vi "SDSU_REgister2Str.vi"(9 "send comment":bool, 10 "Register":T1) -> (1 "fields info":string, 2 "full info":string)   [LabVIEW 2016]
uses:
  SDSU_Register.ctl
  SDSU_RegField.ctl
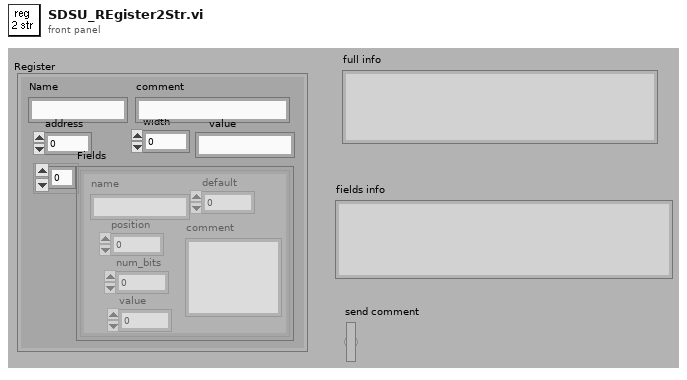
[diagram p1: front panel]
types:
  T1 = typedef "SDSU_Register.ctl" = cluster{"Name":string, "address":i16, "width":i16, "comment":string, "Fields":T2[], "value":string}
  T2 = typedef "SDSU_RegField.ctl" = cluster{"name":string, "position":u16, "num_bits":u16, "default":i16, "comment":string, "value":i32}
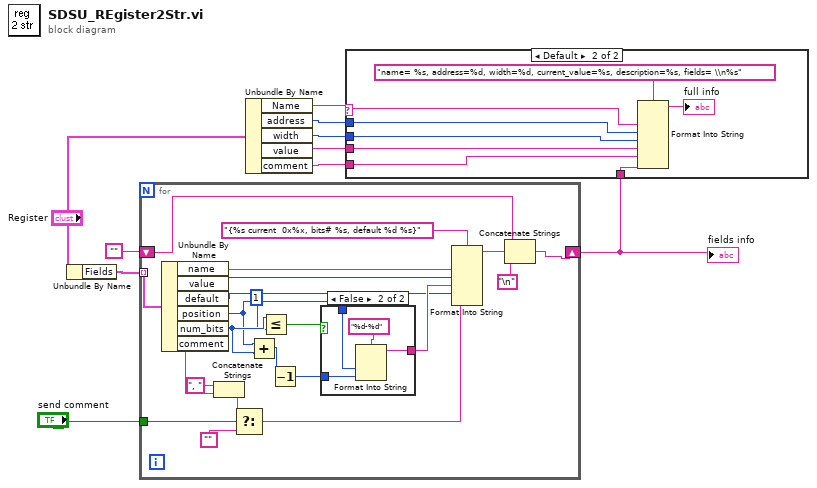
[diagram p0: block diagram]
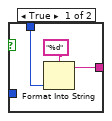
[diagram p3: hidden frame]
diagram:
  n1 = Unbundle By Name("Register") -> ("Fields"=w10:T2[])
  n2 = for {
    tunnel: w10 -> [w32] mode=indexing
    shift-right: [w27] -> w3
    shift-left: "" -> [w26]
    tunnel: "send comment" -> [w17]
    n3 = Unbundle By Name(w32) -> ("name"=w30:string, "value"=w29:i32, "default"=w20:i16, "position"=w23:u16, "num_bits"=w25:u16, "comment"=w14:string)
    n4 = Concatenate Strings(", " ("string"), w14) -> (w12:string)
    n5 = Select(t=w12, s=w17, f="") -> (s? t:f=w15:string)
    n6 = Add(x=w23, y=w25) -> (x+y=w22:u16)
    n7 = Less Or Equal?(x=w25, y=u16 1) -> (x <= y?=w19:bool)
    n8 = Decrement(x=w22) -> (x-1=w11:u16)
    n9 = case shown="False" w19 {
      tunnel: w23 -> [w35 w39]
      tunnel: w11 -> [_ w38]
      tunnel: [w34 w37] -> w21
      frame True {
        n10 = Format Into String(format string="%d", w35) -> (resulting string=w34:string)  [unwired: 2 in, 1 out]
      }
      frame False {
        n11 = Format Into String(format string="%d-%d", w39, w38) -> (resulting string=w37:string)  [unwired: 2 in, 1 out]
      }
    }
    n12 = Format Into String(format string="{%s current  0x%x, bits# %s, default %d %s}", w30, w29, w21, w20, w15) -> (resulting string=w28:string)  [unwired: 2 in, 1 out]
    n13 = Concatenate Strings(w26, w28, "\n") -> (w27:string)
  }
  "fields info" <- w3
  n14 = Unbundle By Name("Register") -> ("Name"=w2:string, "address"=w8:i16, "width"=w7:i16, "value"=w5:string, "comment"=w4:string)
  n15 = case shown="Default" w2 {
    selector: w2 -> [_ w40]
    tunnel: w8 -> [_ w46]
    tunnel: w7 -> [_ w45]
    tunnel: w5 -> [_ w43]
    tunnel: w4 -> [_ w42]
    tunnel: w3 -> [_ w41]
    frame "", " " {
    }
    frame Default {
      n16 = Format Into String(format string="name= %s, address=%d, width=%d, current_value=%s, description=%s, fields= \\n%s", w40, w46, w45, w43, w42, w41) -> (resulting string=→"full info":string)  [unwired: 2 in, 1 out]
    }
  }
